vi "Trigger.vi"() -> ()   [LabVIEW 2016]
uses:
  <vilib>/rvi/Emulation/niFpgaGetClockAttributes.vi
  <vilib>/rvi/Emulation/niFpgaSctlEmulationGetInTimedLoop.vi
  <vilib>/rvi/Emulation/niFpgaEmulationReportErrorSimple.vi
  <vilib>/rvi/eio/common/nirviEmuTemplateMethod_errors.vi
  <vilib>/rvi/Emulation/niFpgaCriticalErrorInLSC.vi
  <vilib>/eio/EIONode/EIONode.xnode
panel:
  in  "Fluoview Delay (ms)":i16=5
  in  "Fluoview Frequency (Hz)":i16=50
  in  "ArenaView Frequency (Hz)":i16=50
  in  "Flyview: Frequency (Hz)":u16=1000
  in  "Duty Cycle (%)":i16=90
  # "Flyception Trigger Settings"
  # "FLYVIEW:"
  # "Falling Edge Triggered / Duty Cycle Low"
  # "Frequency (Hz):"
  # "Duty Cycle (Low) %:"
  # "ARENAVIEW:"
  # "Frequency (Hz):"
  # "FLUOVIEW:"
  # "Frequency (Hz):"
  # "Delay (ms):"
  # "NOTE: All freqencies must be less than loop frequency 10 kHz"
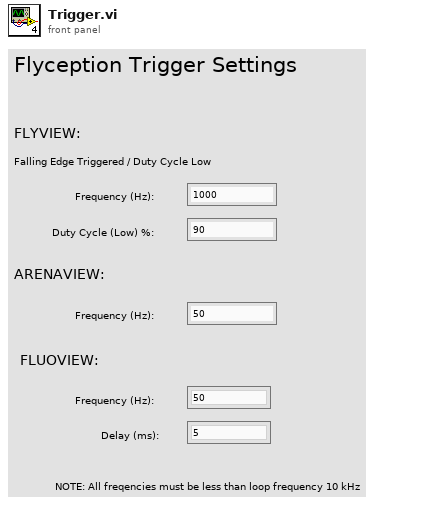
[diagram p1: front panel]
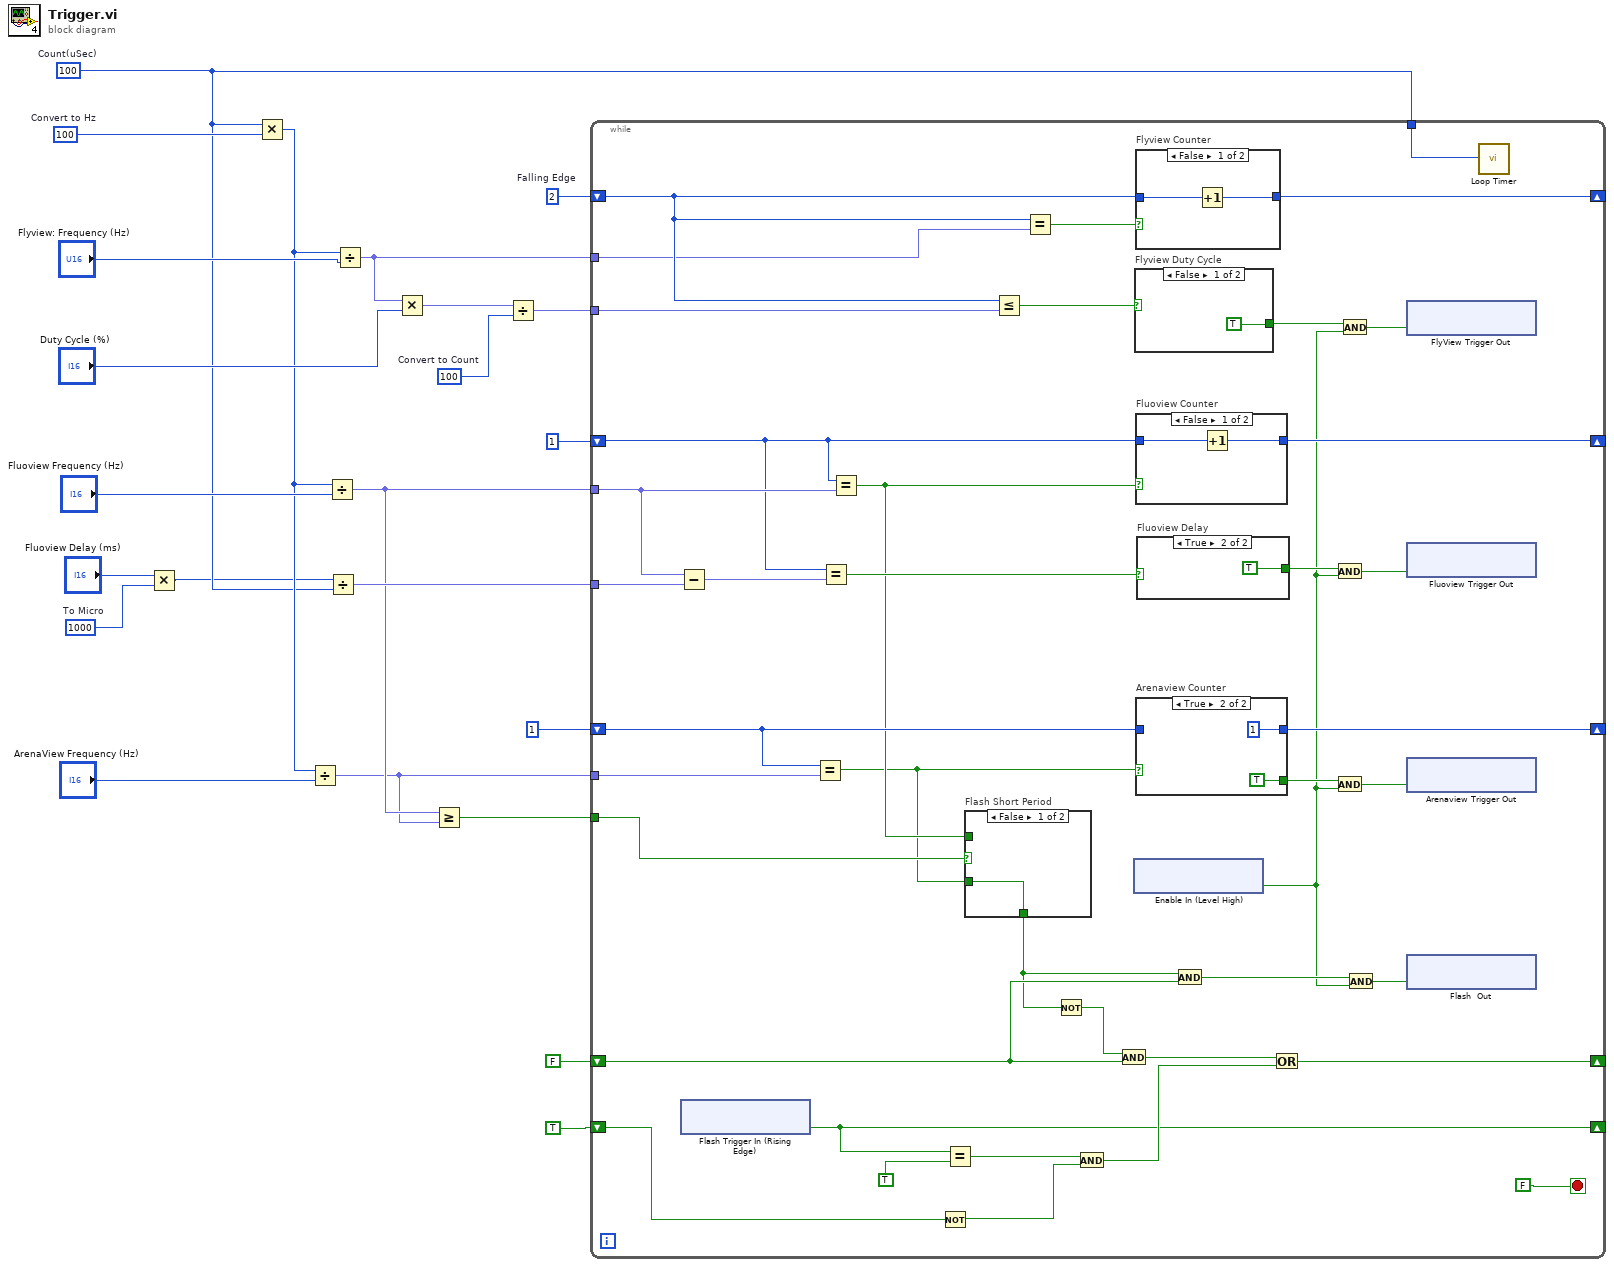
[diagram p0: block diagram]
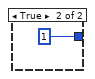
[diagram p3: hidden frame]
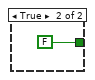
[diagram p4: hidden frame]
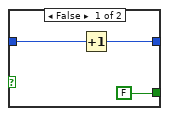
[diagram p5: hidden frame]
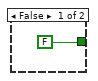
[diagram p6: hidden frame]
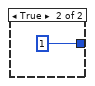
[diagram p7: hidden frame]
diagram:
  w7 = u16 1000  # To Micro
  w14 = u16 100  # Convert to Count
  w19 = u16 100  # Convert to Hz
  w2 = u16 100  # Count(uSec)
  w23 = i16 2  # Falling Edge
  n1 = Multiply(x="Fluoview Delay (ms)", y=w7) -> (x*y=w1:u16)
  n2 = Multiply(x=w2, y=w19) -> (x*y=w9:u16)
  n3 = Divide(x=w9, y="ArenaView Frequency (Hz)") -> (x/y=w4:fxp<+,16,16>)
  n4 = Divide(x=w9, y="Fluoview Frequency (Hz)") -> (x/y=w5:fxp<+,16,16>)
  n5 = Divide(x=w1, y=w2) -> (x/y=w6:fxp<+,16,16>)
  n6 = Divide(x=w9, y="Flyview: Frequency (Hz)") -> (x/y=w17:fxp<+,16,16>)
  n7 = Multiply(x=w17, y="Duty Cycle (%)") -> (x*y=w15:fxp<+/-,32,32>)
  n8 = Greater Or Equal?(x=w5, y=w4) -> (x >= y?=w3:bool)
  n9 = Divide(x=w15, y=w14) -> (x/y=w13:fxp<+,16,16>)
  n10 = while {
    shift-right: [w63] -> _
    shift-left: w23 -> [w59]
    shift-right: [w62] -> _
    shift-left: i16 1 -> [w57]
    shift-right: [w58] -> _
    shift-left: i16 1 -> [w40]
    shift-right: [w47] -> _
    shift-left: TRUE -> [w50]
    shift-right: [w51] -> _
    shift-left: FALSE -> [w48]
    tunnel: w2 -> [w46]
    tunnel: w17 -> [w45]
    tunnel: w13 -> [w44]
    tunnel: w4 -> [w43]
    tunnel: w5 -> [w42]
    tunnel: w6 -> [w41]
    tunnel: w3 -> [w37]
    stop <- FALSE stop-if-true
    n11 = Subtract(x=w42, y=w41) -> (x-y=w39:fxp<+/-,17,17>)
    n12 = xnode "Flash Trigger In (Rising Edge)"() -> ("ConnectorC/DIO7"=w47:bool)  [unwired: 1 in, 1 out]
    n13 = Equal?(x=w57, y=w43) -> (x = y?=w35:bool)
    n14 = Equal?(x=w40, y=w39) -> (x = y?=w38:bool)
    n15 = Equal?(x=w40, y=w42) -> (x = y?=w36:bool)
    n16 = Not(x=w50) -> (.not. x?=w49:bool)
    n17 = Equal?(x=w47, y=TRUE) -> (x = y?=w55:bool)
    n18 = case "Flash Short Period" shown="False" w37 {
      tunnel: w36 -> [_ w65]
      tunnel: w35 -> [w64 _]
      tunnel: [w64 w65] -> w34
      frame False {
      }
      frame True {
      }
    }
    n19 = Less Or Equal?(x=w59, y=w44) -> (x <= y?=w60:bool)
    n20 = Equal?(x=w59, y=w45) -> (x = y?=w61:bool)
    n21 = Not(x=w34) -> (.not. x?=w53:bool)
    n22 = And(x=w55, y=w49) -> (x .and. y?=w54:bool)
    n23 = And(x=w53, y=w48) -> (x .and. y?=w52:bool)
    n24 = xnode "Enable In (Level High)"() -> ("ConnectorC/DIO6"=w25:bool)  [unwired: 1 in, 1 out]
    n25 = case "Flyview Duty Cycle" shown="False" w60 {
      tunnel: [TRUE FALSE] -> w33
      frame False {
      }
      frame True {
      }
    }
    n26 = case "Flyview Counter" shown="False" w61 {
      tunnel: [w78 i16 1] -> w63
      tunnel: w59 -> [w79 _]
      frame False {
        n27 = Increment(x=w79) -> (x+1=w78:i16)
      }
      frame True {
      }
    }
    n28 = case "Fluoview Counter" shown="False" w36 {
      tunnel: [w66 i16 1] -> w58
      tunnel: w40 -> [w67 _]
      frame False {
        n29 = Increment(x=w67) -> (x+1=w66:i16)
      }
      frame True {
      }
    }
    n30 = case "Arenaview Counter" shown="True" w35 {
      tunnel: [FALSE TRUE] -> w30
      tunnel: [w71 i16 1] -> w62
      tunnel: w57 -> [w72 _]
      frame False {
        n31 = Increment(x=w72) -> (x+1=w71:i16)
      }
      frame True {
      }
    }
    n32 = case "Fluoview Delay" shown="True" w38 {
      tunnel: [FALSE TRUE] -> w31
      frame False {
      }
      frame True {
      }
    }
    n33 = And(x=w34, y=w48) -> (x .and. y?=w29:bool)
    n34 = Or(x=w52, y=w54) -> (x .or. y?=w51:bool)
    n35 = And(x=w31, y=w25) -> (x .and. y?=w28:bool)
    n36 = And(x=w30, y=w25) -> (x .and. y?=w27:bool)
    n37 = And(x=w33, y=w25) -> (x .and. y?=w32:bool)
    n38 = And(x=w29, y=w25) -> (x .and. y?=w26:bool)
    n39 = xnode "FlyView Trigger Out"("ConnectorC/DIO0"=w32) -> ()  [unwired: 1 in, 1 out]
    n40 = xnode "Fluoview Trigger Out"("ConnectorC/DIO1"=w28) -> ()  [unwired: 1 in, 1 out]
    n41 = xnode "Arenaview Trigger Out"("ConnectorC/DIO2"=w27) -> ()  [unwired: 1 in, 1 out]
    n42 = xnode "Flash  Out"("ConnectorC/DIO3"=w26) -> ()  [unwired: 1 in, 1 out]
    n43 = call "Loop Timer"("Count(uSec)"=w46) -> ()  [unwired: 1 out]
  }
